vi "PDE_SpMtrx_BiCG Sym Solver.vi"(6 "termination":cluster{"max iter":i32, "tolerance":dbl}={"max iter"=200, "tolerance"=1e-08}, 8 "error in (no error)":errorcluster, 9 "X0":dbl[](array[numeric]), 10 "RHS":dbl[](array[numeric]), 11 "Sparse Mtrx":T1) -> (0 "error out":errorcluster, 3 "X":dbl[](array[numeric]))   [LabVIEW 2017, in "NI_PDE.lvlib"]
uses:
  <vilib>/gmath/NI_PDE.lvlib
  <vilib>/gmath/pde.llb/Common/PDE_Sparse Mtrx.ctl
  <vilib>/Analysis/baseanly.llb/Real Dot Product.vi
  <vilib>/Analysis/NI_AALBase.lvlib
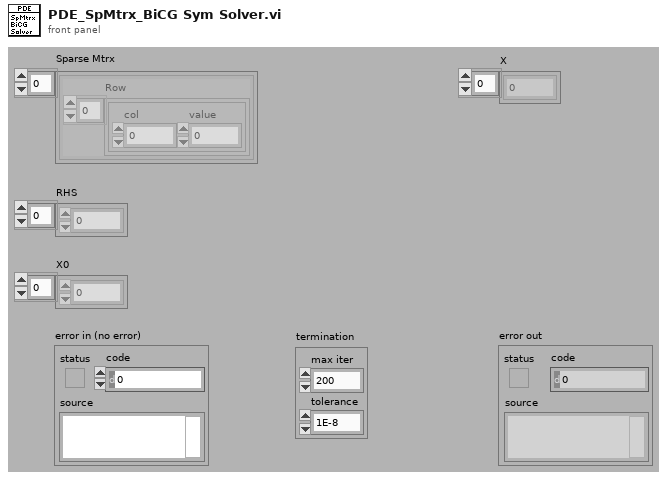
[diagram p1: front panel]
types:
  T1 = typedef "NI_PDE.lvlib/PDE_Sparse Mtrx.ctl" = cluster{"Row":cluster{"col":i32, "value":dbl}[]}[]
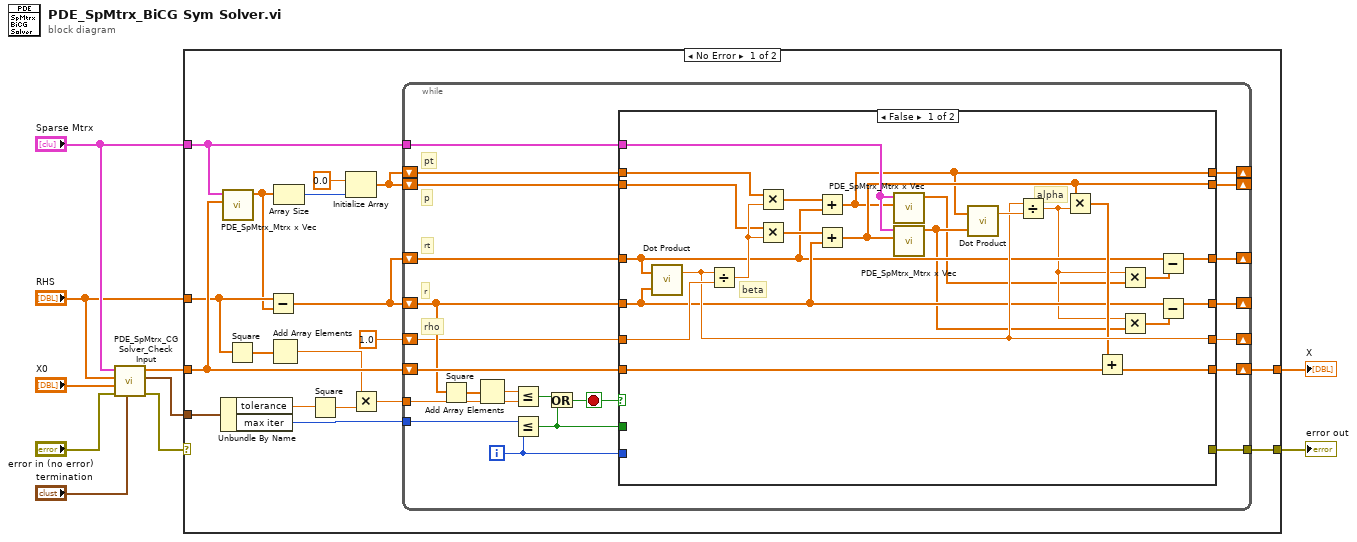
[diagram p0: block diagram]
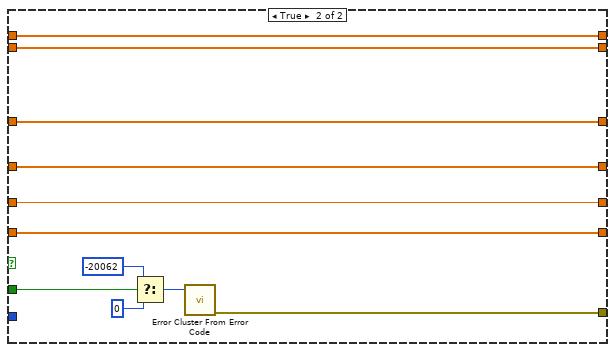
[diagram p2: hidden frame]
diagram:
  n1 = call <vilib>:"PDE_SpMtrx_CG Solver_Check Input.vi"("termination in"="termination", "error in (no error)"="error in (no error)", "X0 In"="X0", "RHS"="RHS", "Sparse Mtrx"="Sparse Mtrx") -> ("error out"=w2:errorcluster, "termination out"=w4:cluster{"max iter":i32, "tolerance":dbl}, "X0 Out"=w3:dbl[])  [unwired: 4 out]
  n2 = case shown="No Error" w2 {
    selector: w2 -> [_ w85]
    tunnel: w4 -> [w28 _]
    tunnel: w3 -> [w18 _]
    tunnel: "Sparse Mtrx" -> [w24 _]
    tunnel: "RHS" -> [w16 _]
    tunnel: [w23 _] -> w10
    tunnel: [w19 w85] -> w9
    frame No Error {
      n3 = Unbundle By Name(w28) -> ("tolerance"=w26:dbl, "max iter"=w27:i32)
      n4 = call <vilib>:"PDE_SpMtrx_Mtrx x Vec.vi"("X"=w18, "Sparse Mtrx"=w24) -> ("Mtrx x X"=w12:dbl[])  [unwired: 9 out]
      n5 = Square(x=w16) -> (x^2=w21:dbl[])
      n6 = Subtract(x=w16, y=w12) -> (x-y=w22:dbl[])
      n7 = Add Array Elements(numeric array=w21) -> (sum=w17:dbl)
      n8 = Array Size(array=w12) -> (size(s)=w11:i32)
      n9 = Square(x=w26) -> (x^2=w20:dbl)
      n10 = Initialize Array(0.0 ("element"), w11) -> (w13:dbl[])
      n11 = Multiply(x=w17, y=w20) -> (x*y=w25:dbl)
      n12 = while {
        tunnel: w25 -> [w50]
        shift-right: [w46] -> w23
        shift-left: w18 -> [w47]
        shift-right: [w41] -> _
        shift-left: w22 -> [w36]
        tunnel: w27 -> [w49]
        tunnel: w24 -> [w42]
        shift-right: [w43] -> _
        shift-left: w22 -> [w44]
        tunnel: [w38] -> w19
        shift-right: [w31] -> _
        shift-left: 1.0 ("Numeric") -> [w34]
        shift-right: [w30] -> _
        shift-left: w13 -> [w33]
        shift-right: [w29] -> _
        shift-left: w13 -> [w32]
        i -> [w45]
        stop <- w40 stop-if-true
        # "pt"
        # "p"
        # "rho"
        # "rt"
        # "r"
        n13 = Square(x=w36) -> (x^2=w37:dbl[])
        n14 = Add Array Elements(numeric array=w37) -> (sum=w35:dbl)
        n15 = Less Or Equal?(x=w35, y=w50) -> (x <= y?=w48:bool)
        n16 = Less Or Equal?(x=w49, y=w45) -> (x <= y?=w39:bool)
        n17 = Or(x=w48, y=w39) -> (x .or. y?=w40:bool)
        n18 = case shown="False" w40 {
          tunnel: w47 -> [w65 w83]
          tunnel: [w64 w83] -> w46
          tunnel: w45 -> [_ _]
          tunnel: w36 -> [w61 w82]
          tunnel: w44 -> [w58 w84]
          tunnel: [w57 w84] -> w43
          tunnel: w42 -> [w69 _]
          tunnel: [w60 w82] -> w41
          tunnel: w39 -> [_ w81]
          tunnel: [_ w77] -> w38
          tunnel: w34 -> [w73 w76]
          tunnel: w33 -> [w63 w74]
          tunnel: w32 -> [w68 w75]
          tunnel: [w66 w76] -> w31
          tunnel: [w54 w74] -> w30
          tunnel: [w53 w75] -> w29
          frame False {
            # "alpha"
            # "beta"
            n19 = call-poly <vilib>:"Dot Product.vi"("Y Vector"=w61, "X Vector"=w58) -> ("X * Y"=w66:dbl)  [unwired: 1 out]
            n20 = Divide(x=w66, y=w73) -> (x/y=w71:dbl)
            n21 = Multiply(x=w68, y=w71) -> (x*y=w70:dbl[])
            n22 = Multiply(x=w63, y=w71) -> (x*y=w72:dbl[])
            n23 = Add(x=w70, y=w58) -> (x+y=w53:dbl[])
            n24 = Add(x=w72, y=w61) -> (x+y=w54:dbl[])
            n25 = call <vilib>:"PDE_SpMtrx_Mtrx x Vec.vi"("X"=w53, "Sparse Mtrx"=w69) -> ("Mtrx x X"=w51:dbl[])  [unwired: 9 out]
            n26 = call <vilib>:"PDE_SpMtrx_Mtrx x Vec.vi"("X"=w54, "Sparse Mtrx"=w69) -> ("Mtrx x X"=w52:dbl[])  [unwired: 9 out]
            n27 = call-poly <vilib>:"Dot Product.vi"("Y Vector"=w52, "X Vector"=w53) -> ("X * Y"=w67:dbl)  [unwired: 1 out]
            n28 = Divide(x=w66, y=w67) -> (x/y=w56:dbl)
            n29 = Multiply(x=w54, y=w56) -> (x*y=w62:dbl[])
            n30 = Add(x=w62, y=w65) -> (x+y=w64:dbl[])
            n31 = Multiply(x=w56, y=w51) -> (x*y=w55:dbl[])
            n32 = Multiply(x=w56, y=w52) -> (x*y=w59:dbl[])
            n33 = Subtract(x=w58, y=w55) -> (x-y=w57:dbl[])
            n34 = Subtract(x=w61, y=w59) -> (x-y=w60:dbl[])
          }
          frame True {
            n35 = Select(t=-20062, s=w81, f=0) -> (s? t:f=w78:i32)
            n36 = call <vilib>:"Error Cluster From Error Code.vi"("error code (0)"=w78) -> ("error out"=w77:errorcluster)  [unwired: 2 in, 6 out]
          }
        }
      }
    }
    frame Error {
    }
  }
  "X" <- w10
  "error out" <- w9
